vi "CoboltLaser_TECTempsGet.vi"(0 "ComPort":refnum<visa-resource-name>, 3 "CheckResponse":bool=TRUE, 7 "error in (no error)":errorcluster) -> (20 "ComPortOut":refnum<visa-resource-name>, 21 "TEC tempeartures":dbl[](array[numeric]), 27 "error out":errorcluster)   [LabVIEW 2012, in "Cobolt.lvclass"]
doc: "Use this template to build a VI to use as a subVI."
uses:
  Template/Cobolt.lvclass
panel:
  out "ResponseOK":bool
  out "Response":string
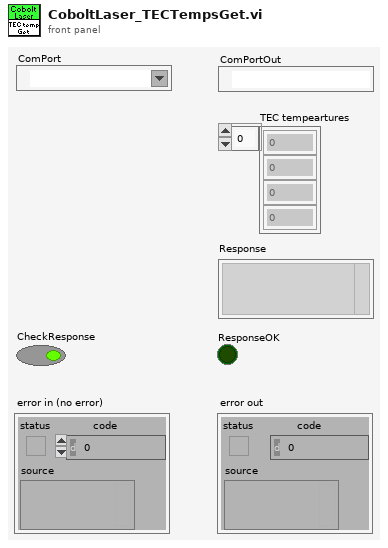
[diagram p1: front panel]
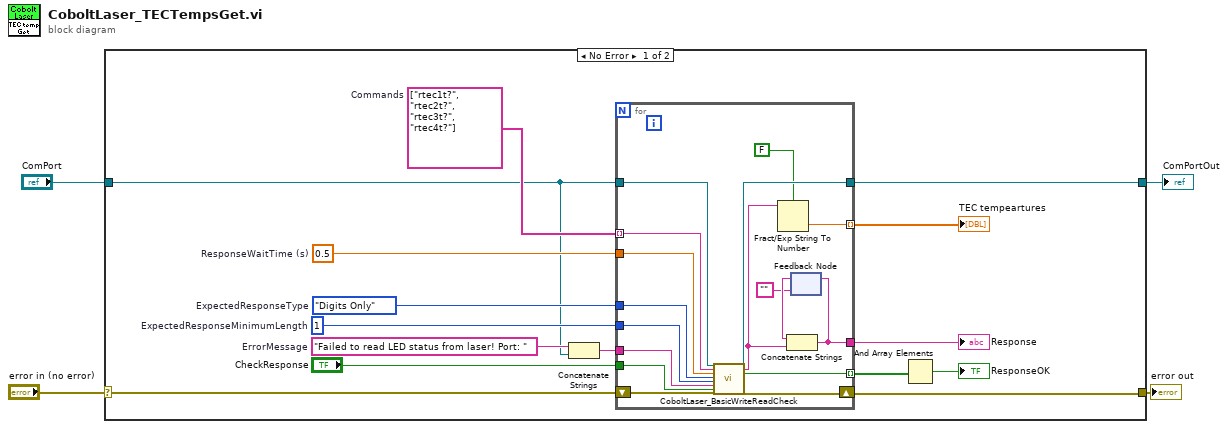
[diagram p0: block diagram]
diagram:
  n1 = case shown="No Error" "error in (no error)" {
    selector: "error in (no error)" -> [w19 w38]
    tunnel: [w18 w38] -> w3
    tunnel: "ComPort" -> [w6 w37]
    tunnel: [w5 w37] -> w1
    frame No Error {
      w11 = string[] ["rtec1t?", "rtec2t?", "rtec3t?", "rtec4t?"]  # Commands
      w15 = 1  # ExpectedResponseMinimumLength
      w16 = enum16{"Any", "Digits Only", "Non-Digits Only"}."Digits Only"  # ExpectedResponseType
      w17 = 0.5  # ResponseWaitTime (s)
      w13 = "Failed to read LED status from laser! Port: "  # ErrorMessage
      n2 = Concatenate Strings(w13, w6) -> (w12:string)
      n3 = for {
        tunnel: w17 -> [w34]
        tunnel: w11 -> [w33] mode=indexing
        tunnel: w16 -> [w32]
        tunnel: w15 -> [w31]
        tunnel: "CheckResponse" -> [w30]
        tunnel: [w29] -> w5
        tunnel: [w28] -> w10 mode=indexing
        tunnel: w12 -> [w27]
        tunnel: w6 -> [w26]
        shift-right: [w35] -> w18
        shift-left: w19 -> [w36]
        tunnel: [w25] -> w7 mode=indexing
        tunnel: [w22] -> w8
        n4 = call "CoboltLaser_BasicWriteReadCheck.vi"("ComPort"=w26, "Command"=w33, "ResponseWaitTime (s)"=w34, "ExpectedResponseType"=w32, "ExpectedResponseMinimumLength"=w31, "ErrorMessage"=w27, "CheckResponse"=w30, "error in (no error)"=w36) -> ("ComPortOut"=w29:refnum<visa-resource-name>, "Response"=w24:string, "ResponseOK"=w28:bool, "error out"=w35:errorcluster)  [unwired: 16 in]
        n5 = Fract/Exp String To Number(use system decimal point (T)=FALSE, string=w24) -> (number=w25:dbl)  [unwired: 2 in, 1 out]
        n6 = feedback #1("") -> (w23:string)
        n7 = Concatenate Strings(w23, w24) -> (w22:string)
        n8 = feedback-in #1(w22) -> ()
      }
      "Response" <- w8
      "TEC tempeartures" <- w7
      n9 = And Array Elements(Boolean array=w10) -> (logical AND=→"ResponseOK":bool)
    }
    frame Error {
    }
  }
  "error out" <- w3
  "ComPortOut" <- w1
